vi "Score_For_Direction.vi"(8 "error in (no error)":errorcluster, 9 "Desired Floor":i32, 10 "Hall Up/Down":T1, 11 "Up/Down/Idle":T1) -> (0 "error out":errorcluster, 3 "Score":i32)   [LabVIEW 2026]
uses:
  Controls/Motion_Status_Enum.ctl
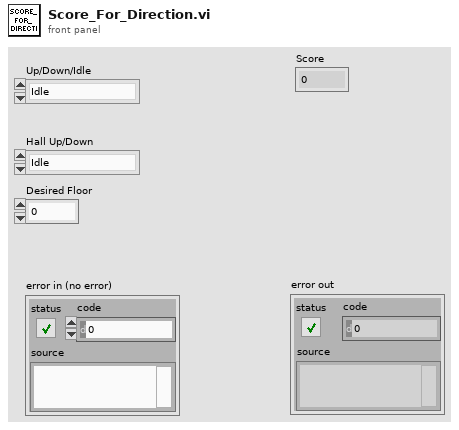
[diagram p1: front panel]
types:
  T1 = typedef "Motion_Status_Enum.ctl" = enum16{"Idle", "Up", "Down"}
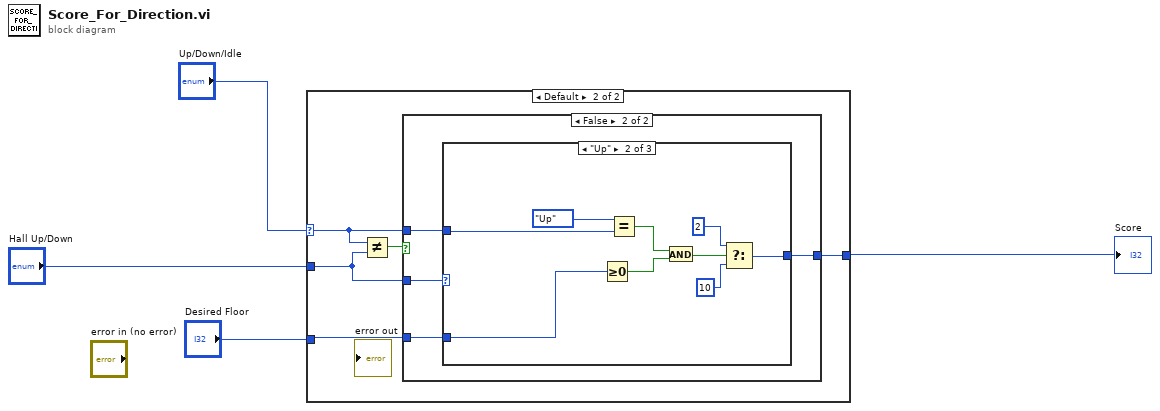
[diagram p0: block diagram]
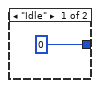
[diagram p2: hidden frame]
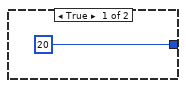
[diagram p3: hidden frame]
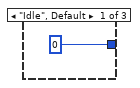
[diagram p4: hidden frame]
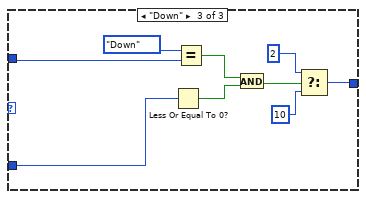
[diagram p5: hidden frame]
diagram:
  n1 = case shown="Default" "Up/Down/Idle" {
    selector: "Up/Down/Idle" -> [_ w6]
    tunnel: "Hall Up/Down" -> [_ w8]
    tunnel: "Desired Floor" -> [_ w7]
    tunnel: [0 w9] -> w2
    frame "Idle" {
    }
    frame Default {
      n2 = Not Equal?(x=w6, y=w8) -> (x != y?=w10:bool)
      n3 = case shown="False" w10 {
        tunnel: [20 w13] -> w9
        tunnel: w8 -> [_ w15]
        tunnel: w7 -> [_ w14]
        tunnel: w6 -> [_ w12]
        frame True {
        }
        frame False {
          n4 = case shown="\"Up\"" w15 {
            tunnel: [0 ("t") w19 w28] -> w13
            tunnel: w14 -> [_ w18 w27]
            tunnel: w12 -> [_ w17 w26]
            frame "Idle", Default {
            }
            frame "Up" {
              n5 = Greater Or Equal To 0?(x=w18) -> (x >= 0?=w23:bool)
              n6 = Equal?(x=Motion_Status_Enum."Up" ("value"), y=w17) -> (x = y?=w24:bool)
              n7 = And(x=w24, y=w23) -> (x .and. y?=w20:bool)
              n8 = Select(t=2, s=w20, f=10 ("t")) -> (s? t:f=w19:i32)
            }
            frame "Down" {
              n9 = Less Or Equal To 0?(x=w27) -> (x <= 0?=w32:bool)
              n10 = Equal?(x=Motion_Status_Enum."Down" ("value"), y=w26) -> (x = y?=w33:bool)
              n11 = And(x=w33, y=w32) -> (x .and. y?=w29:bool)
              n12 = Select(t=2, s=w29, f=10 ("t")) -> (s? t:f=w28:i32)
            }
          }
        }
      }
    }
  }
  "Score" <- w2
